vi "UtilityLib.set colors of panel to defaults.vi"(0 "Front Panel":refnum<vi>, 1 "setBoolIndicators?":bool, 5 "error in (no error)":errorcluster) -> (19 "error out":errorcluster)   [LabVIEW 2015, in "UtilityLib.lvlib"]
doc: "Sets the color of the front panel (to which we get the reference) elements to default values. The intention of this routine is to set the color of all front panels to common default values to provide a common look and feel.\n\nJust call this routine as the first VI when you execute a panel.\n\nHow to get a front panel reference\nFuntcionPallete -> Application Control -> PropertyNode -> Select Class: VI Server-VI-VI ->Property->Front Panel"
uses:
  UtilityLib.lvlib
  UtilityLib.valueStatus.ctl
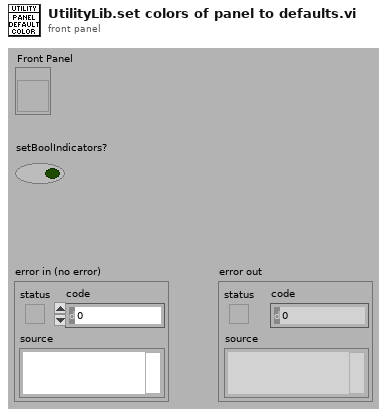
[diagram p1: front panel]
types:
  T1 = typedef "UtilityLib.lvlib/UtilityLib.valueStatus.ctl" = enum16{"no info available", "stand by/off", "on", "warning", "alarm/malfunction", "not implemented", "user action required", "important information", "system default", "control default", "indicator default", "button default"}
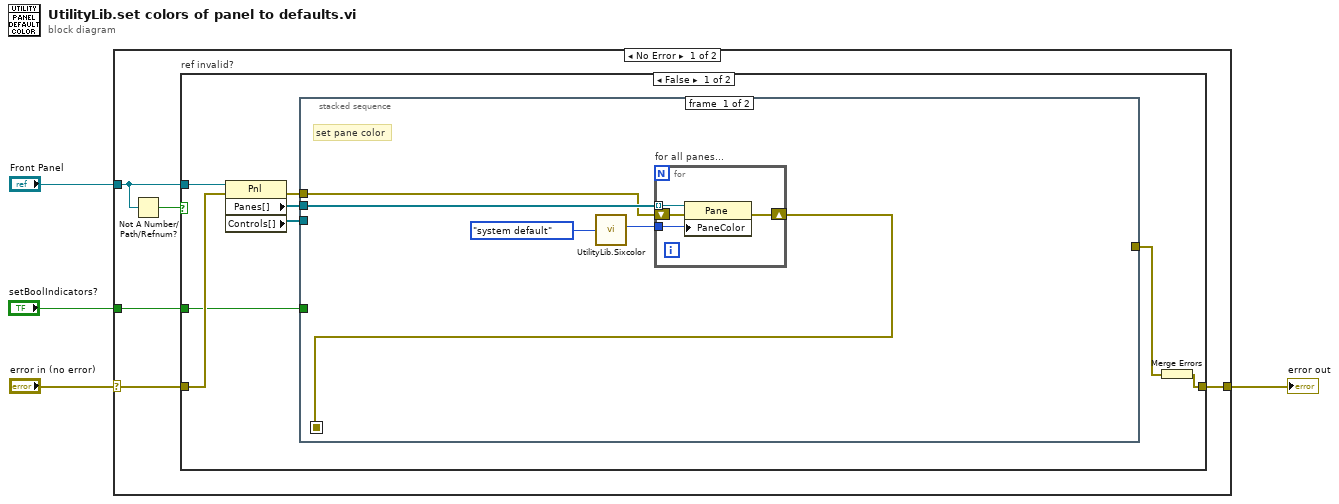
[diagram p0: block diagram]
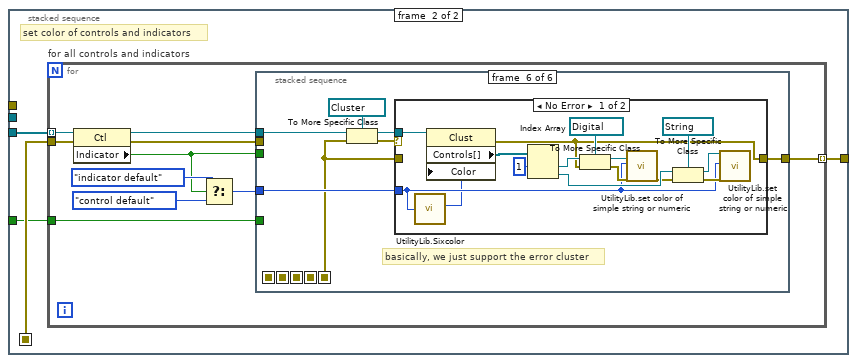
[diagram p2: hidden frame]
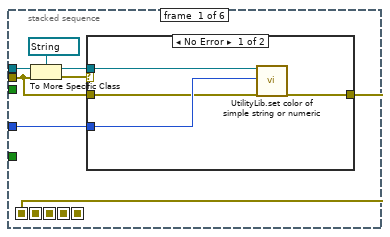
[diagram p3: hidden frame]
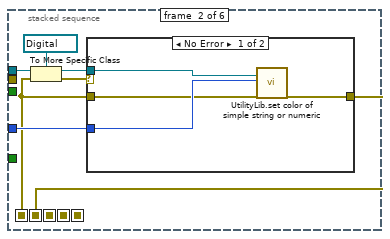
[diagram p5: hidden frame]
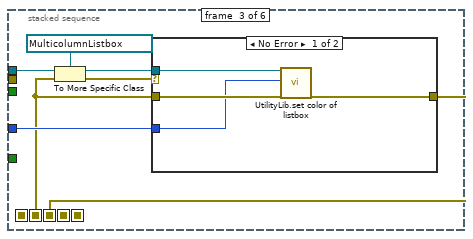
[diagram p7: hidden frame]
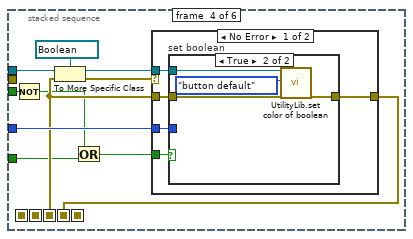
[diagram p9: hidden frame]
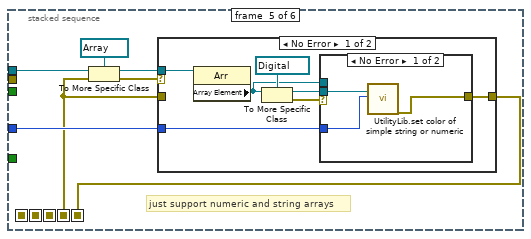
[diagram p12: hidden frame]
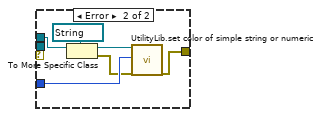
[diagram p13: hidden frame]
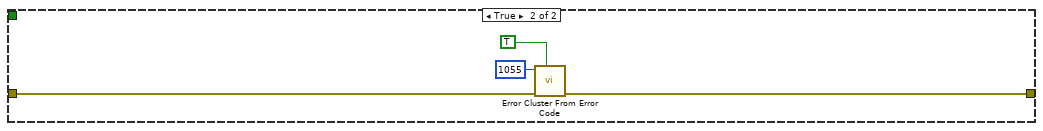
[diagram p16: hidden frame]
diagram:
  n1 = case shown="No Error" "error in (no error)" {
    selector: "error in (no error)" -> [w9 w150]
    tunnel: [w6 w150] -> w1
    tunnel: "Front Panel" -> [w8 _]
    tunnel: "setBoolIndicators?" -> [w5 _]
    frame No Error {
      n2 = Not A Number/Path/Refnum?(number/path/refnum=w8) -> (NaN/Path/Refnum?=w7:bool)
      n3 = case "ref invalid?" shown="False" w7 {
        tunnel: w8 -> [w17 _]
        tunnel: w9 -> [w16 w149]
        tunnel: [w10 w146] -> w6
        tunnel: w5 -> [w12 _]
        frame False {
          n4 = property class="Pnl"(reference=w17, error in=w16) -> (error out=w14:errorcluster, "Panes[]"=w15:refnum<vi>[], "Controls[]"=w13:refnum<vi>[])  [unwired: 1 out]
          n5 = stacked-sequence {
            seq-local: [w20 _] -> [_ w29]
            tunnel: w15 -> [w19 _]
            tunnel: w14 -> [w18 _]
            tunnel: w13 -> [_ w30]
            tunnel: w12 -> [_ w28]
            tunnel: [_ w27] -> w11
            frame #0 {
              # "set pane color"
              n6 = call "UtilityLib.Sixcolor.vi"("State"=UtilityLib.valueStatus."system default") -> ("elementBackground"=w22:u32)  [unwired: 2 in, 3 out]
              n7 = for "for all panes..." {
                tunnel: w19 -> [w26] mode=indexing
                tunnel: w22 -> [w25]
                shift-right: [w23] -> w20
                shift-left: w18 -> [w24]
                n8 = property class="Pane"(reference=w26, error in=w24, "PaneColor"=w25) -> (error out=w23:errorcluster)  [unwired: 1 out]
              }
            }
            frame #1 {
              # "set color of controls and indicators"
              n9 = for "for all controls and indicators" {
                tunnel: w30 -> [w40] mode=indexing
                tunnel: w28 -> [w32]
                tunnel: w29 -> [w39]
                tunnel: [w31] -> w27 mode=indexing
                n10 = property class="Ctl"(reference=w40, error in=w39) -> (reference out=w38:refnum<vi>, error out=w34:errorcluster, "Indicator"=w33:bool)
                n11 = Select(t=UtilityLib.valueStatus."indicator default" ("valueStatus"), s=w33, f=UtilityLib.valueStatus."control default") -> (s? t:f=w35:T1)
                n12 = stacked-sequence {
                  seq-local: [w43 _ _ _ _ _] -> [_ w54 _ _ _ _]
                  seq-local: [_ w55 _ _ _ _] -> [_ _ w67 _ _ _]
                  seq-local: [_ _ w66 _ _ _] -> [_ _ _ w83 _ _]
                  seq-local: [_ _ _ w78 _ _] -> [_ _ _ _ w101 _]
                  seq-local: [_ _ _ _ w100 _] -> [_ _ _ _ _ w125]
                  tunnel: w38 -> [w45 w57 w69 w85 w103 w127]
                  tunnel: w35 -> [w44 w56 w68 w84 w102 w126]
                  tunnel: w34 -> [w42 _ _ _ _ _]
                  tunnel: w33 -> [_ _ _ w82 _ _]
                  tunnel: w32 -> [_ _ _ w80 _ _]
                  tunnel: [_ _ _ _ _ w123] -> w31
                  frame #0 {
                    n13 = To More Specific Class(target class=refnum<vi> refnum ("simpleString"), reference=w45, error in=w42) -> (specific class reference=w46:refnum<vi>, error out=w47:errorcluster)
                    n14 = case shown="No Error" w47 {
                      tunnel: w46 -> [w48 _]
                      tunnel: w44 -> [w51 _]
                      tunnel: [w50 w52] -> w43
                      tunnel: w42 -> [w49 w52]
                      frame No Error {
                        n15 = call "UtilityLib.set color of simple string or numeric.vi"("simpleString"=w48, "valueStatus"=w51, "error in (no error)"=w49) -> ("error out"=w50:errorcluster)  [unwired: 16 in]
                      }
                      frame Error {
                      }
                    }
                  }
                  frame #1 {
                    n16 = To More Specific Class(target class=refnum<vi> refnum ("simpleNumeric"), reference=w57, error in=w54) -> (specific class reference=w58:refnum<vi>, error out=w59:errorcluster)
                    n17 = case shown="No Error" w59 {
                      tunnel: w58 -> [w62 _]
                      tunnel: w56 -> [w63 _]
                      tunnel: [w61 w64] -> w55
                      tunnel: w54 -> [w60 w64]
                      frame No Error {
                        n18 = call "UtilityLib.set color of simple string or numeric.vi"("simpleNumeric"=w62, "valueStatus"=w63, "error in (no error)"=w60) -> ("error out"=w61:errorcluster)  [unwired: 16 in]
                      }
                      frame Error {
                      }
                    }
                  }
                  frame #2 {
                    n19 = To More Specific Class(target class=refnum<vi> refnum ("listboxRef"), reference=w69, error in=w67) -> (specific class reference=w70:refnum<vi>, error out=w71:errorcluster)
                    n20 = case shown="No Error" w71 {
                      tunnel: w70 -> [w73 _]
                      tunnel: w68 -> [w72 _]
                      tunnel: [w75 w76] -> w66
                      tunnel: w67 -> [w74 w76]
                      frame No Error {
                        n21 = call "UtilityLib.set color of listbox.vi"("listboxRef"=w73, "valueStatus"=w72, "error in (no error)"=w74) -> ("error out"=w75:errorcluster)  [unwired: 16 in]
                      }
                      frame Error {
                      }
                    }
                  }
                  frame #3 {
                    n22 = Not(x=w82) -> (.not. x?=w81:bool)
                    n23 = To More Specific Class(target class=refnum<vi> refnum ("button"), reference=w85, error in=w83) -> (specific class reference=w86:refnum<vi>, error out=w87:errorcluster)
                    n24 = Or(x=w81, y=w80) -> (x .or. y?=w79:bool)
                    n25 = case shown="No Error" w87 {
                      tunnel: w86 -> [w89 _]
                      tunnel: w84 -> [w92 _]
                      tunnel: [w91 w98] -> w78
                      tunnel: w83 -> [w90 w98]
                      tunnel: w79 -> [w88 _]
                      frame No Error {
                        n26 = case "set boolean" shown="True" w88 {
                          tunnel: w92 -> [_ _]
                          tunnel: [w93 w97] -> w91
                          tunnel: w90 -> [w93 w96]
                          tunnel: w89 -> [_ w94]
                          frame False {
                          }
                          frame True {
                            n27 = call "UtilityLib.set color of boolean.vi"("button"=w94, "valueStatus"=UtilityLib.valueStatus."button default", "error in (no error)"=w96) -> ("error out"=w97:errorcluster)  [unwired: 16 in]
                          }
                        }
                      }
                      frame Error {
                      }
                    }
                  }
                  frame #4 {
                    # "just support numeric and string arrays"
                    n28 = To More Specific Class(target class=refnum<vi> refnum ("numArrayType"), reference=w103, error in=w101) -> (specific class reference=w104:refnum<vi>, error out=w105:errorcluster)
                    n29 = case shown="No Error" w105 {
                      tunnel: w104 -> [w109 _]
                      tunnel: w102 -> [w111 _]
                      tunnel: [w110 w122] -> w100
                      tunnel: w101 -> [_ w122]
                      frame No Error {
                        n30 = property class="Arr"(reference=w109) -> ("Array Element"=w106:refnum<vi>)  [unwired: 1 in, 2 out]
                        n31 = To More Specific Class(target class=refnum<vi> refnum ("simpleNumeric"), reference=w106) -> (specific class reference=w112:refnum<vi>, error out=w107:errorcluster)  [unwired: 1 in]
                        n32 = case shown="No Error" w107 {
                          tunnel: w112 -> [w115 _]
                          tunnel: w111 -> [w114 w118]
                          tunnel: [w113 w117] -> w110
                          tunnel: w106 -> [_ w121]
                          frame No Error {
                            n33 = call "UtilityLib.set color of simple string or numeric.vi"("simpleNumeric"=w115, "valueStatus"=w114) -> ("error out"=w113:errorcluster)  [unwired: 17 in]
                          }
                          frame Error {
                            n34 = To More Specific Class(target class=refnum<vi> refnum ("simpleString"), reference=w121) -> (specific class reference=w119:refnum<vi>, error out=w116:errorcluster)  [unwired: 1 in]
                            n35 = call "UtilityLib.set color of simple string or numeric.vi"("simpleString"=w119, "valueStatus"=w118, "error in (no error)"=w116) -> ("error out"=w117:errorcluster)  [unwired: 16 in]
                          }
                        }
                      }
                      frame Error {
                      }
                    }
                  }
                  frame #5 {
                    # "basically, we just support the error cluster"
                    n36 = To More Specific Class(target class=refnum<vi> refnum ("simpleNumeric"), reference=w127, error in=w125) -> (specific class reference=w128:refnum<vi>, error out=w129:errorcluster)
                    n37 = case shown="No Error" w129 {
                      tunnel: w128 -> [w144 _]
                      tunnel: w126 -> [w132 _]
                      tunnel: [w133 w145] -> w123
                      tunnel: w125 -> [_ w145]
                      frame No Error {
                        n38 = call "UtilityLib.Sixcolor.vi"("State"=w132) -> ("elementBackground"=w131:u32)  [unwired: 2 in, 3 out]
                        n39 = property class="Clust"(reference=w144, "Color"=w131) -> (error out=w133:errorcluster, "Controls[]"=w143:refnum<vi>[])  [unwired: 1 in, 1 out]
                        n40 = Index Array(array=w143, index #1=1 ("index")) -> (element #1=w141:refnum<vi>, element #2=w140:refnum<vi>)  [unwired: 1 in]
                        n41 = To More Specific Class(target class=refnum<vi> refnum ("simpleNumeric"), reference=w141, error in=w133) -> (specific class reference=w139:refnum<vi>, error out=w135:errorcluster)
                        n42 = call "UtilityLib.set color of simple string or numeric.vi"("simpleNumeric"=w139, "valueStatus"=w132, "error in (no error)"=w135) -> ("error out"=w130:errorcluster)  [unwired: 16 in]
                        n43 = To More Specific Class(target class=refnum<vi> refnum ("simpleString"), reference=w140, error in=w130) -> (specific class reference=w138:refnum<vi>, error out=w134:errorcluster)
                        n44 = call "UtilityLib.set color of simple string or numeric.vi"("simpleString"=w138, "valueStatus"=w132, "error in (no error)"=w134) -> ()  [unwired: 16 in, 1 out]
                      }
                      frame Error {
                      }
                    }
                  }
                }
              }
            }
          }
          n45 = Merge Errors(w11) -> (w10:errorcluster)
        }
        frame True {
          n46 = call <vilib>:"Error Cluster From Error Code.vi"("show call chain? (False)"=TRUE, "error in (no error)"=w149, "error code (0)"=1055) -> ("error out"=w146:errorcluster)  [unwired: 6 in]
        }
      }
    }
    frame Error {
    }
  }
  "error out" <- w1
